vi "Update Value.vi"(6 "Time":dbl, 8 "error in (no error)":errorcluster, 11 "ImageButtonControl in":refnum<class "ImageButtonControl.lvclass">) -> (0 "error out":errorcluster, 1 "Update":bool, 2 "Value":variant, 3 "ImageButtonControl out":refnum<class "ImageButtonControl.lvclass">)   [LabVIEW 2020, in "VolatusGUIElements.lvlib" / "ImageButtonControl.lvclass"]
uses:
  ImageButtonControl.lvclass
  ImageButtonControl.lvclass/ImageButtonControl.ctl
  lv-vecto/Vecto/Channel DBL/Channel DBL.lvclass/Channel DBL.ctl
  lv-vecto/Vecto/Group DBL/Value by Index.vi
  lv-vecto/Vecto/Channel DBL/Channel DBL.lvclass
  lv-vecto/Vecto/Vecto.lvlib
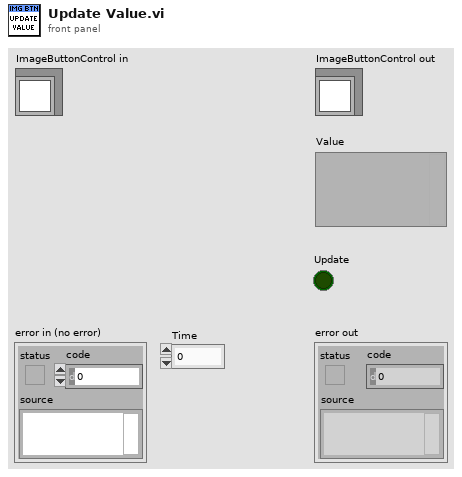
[diagram p1: front panel]
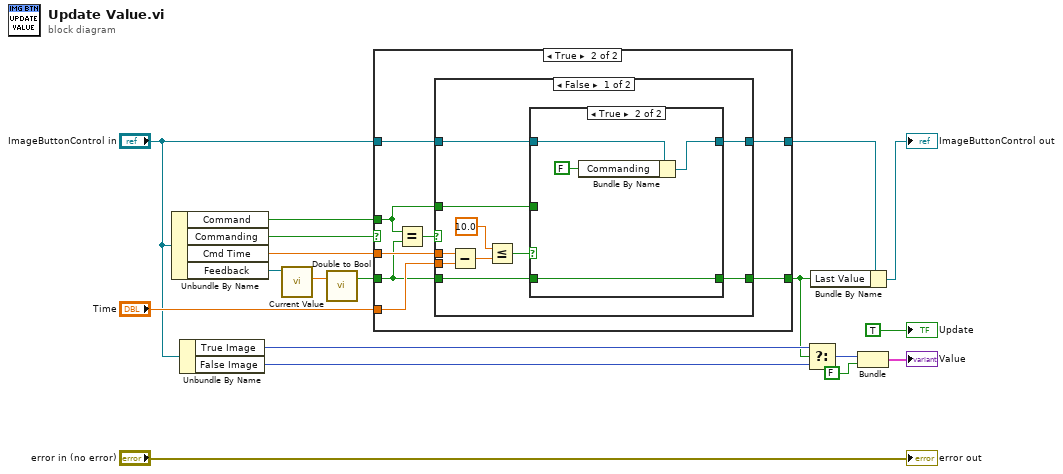
[diagram p0: block diagram]
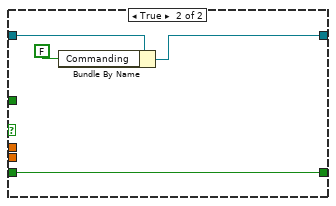
[diagram p4: hidden frame]
diagram:
  n1 = Unbundle By Name("ImageButtonControl in") -> ("Command"=w13:bool, "Commanding"=w17:bool, "Cmd Time"=w15:dbl, "Feedback"=w18:refnum<class "Channel DBL.lvclass">)
  n2 = Unbundle By Name("ImageButtonControl in") -> ("True Image"=w6:picture, "False Image"=w5:picture)
  n3 = call "Current Value.vi"("Channel in"=w18) -> ("Scaled"=w16:dbl)  [unwired: 6 in, 4 out]
  n4 = call "Double to Bool.vi"("Double"=w16) -> ("Bool"=w14:bool)  [unwired: 2 in]
  n5 = case shown="True" w17 {
    tunnel: w14 -> [w20 w25]
    tunnel: w15 -> [_ w28]
    tunnel: "Time" -> [_ w27]
    tunnel: w13 -> [_ w21]
    tunnel: "ImageButtonControl in" -> [w19 w24]
    tunnel: [w19 w23] -> w12
    tunnel: [w20 w22] -> w1
    frame False {
    }
    frame True {
      n6 = Equal?(x=w21, y=w25) -> (x = y?=w26:bool)
      n7 = case shown="False" w26 {
        tunnel: w28 -> [w38 _]
        tunnel: w27 -> [w37 _]
        tunnel: w25 -> [w31 w45]
        tunnel: w24 -> [w33 w48]
        tunnel: [w32 w46] -> w23
        tunnel: [w29 w45] -> w22
        tunnel: w21 -> [w30 _]
        frame False {
          n8 = Subtract(x=w38, y=w37) -> (x-y=w36:dbl)
          n9 = Less Or Equal?(x=10.0, y=w36) -> (x <= y?=w34:bool)
          n10 = case shown="True" w34 {
            tunnel: w33 -> [w39 w44]
            tunnel: [w39 w42] -> w32
            tunnel: w31 -> [_ w41]
            tunnel: w30 -> [w40 _]
            tunnel: [w40 w41] -> w29
            frame False {
            }
            frame True {
              n11 = Bundle By Name(cluster=w44, "Commanding"=FALSE) -> (w42:refnum<class "ImageButtonControl.lvclass">)
            }
          }
        }
        frame True {
          n12 = Bundle By Name(cluster=w48, "Commanding"=FALSE) -> (w46:refnum<class "ImageButtonControl.lvclass">)
        }
      }
    }
  }
  n13 = Select(t=w6, s=w1, f=w5) -> (s? t:f=w4:picture)
  n14 = Bundle By Name(cluster=w12, "Last Value"=w1) -> (→"ImageButtonControl out":refnum<class "ImageButtonControl.lvclass">)
  n15 = Bundle("False Image"=w4, FALSE) -> (→"Value":cluster{"False Image":picture, bool})  [unwired: 1 in]
  "error out" <- "error in (no error)"
  "Update" <- TRUE ("Update")
